vi "Ergetization.vi"(8 "error in (no error)":errorcluster, 11 "Maze in":refnum<class "Maze.lvclass">) -> (0 "error out":errorcluster, 2 "size":i32, 3 "Maze out":refnum<class "Maze.lvclass">)   [LabVIEW 2021, in "Maze.lvclass"]
uses:
  Maze.lvclass
  Maze.lvclass/Maze.ctl
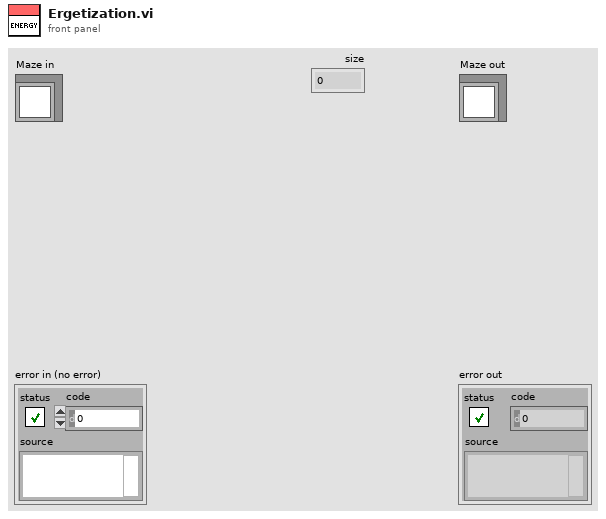
[diagram p1: front panel]
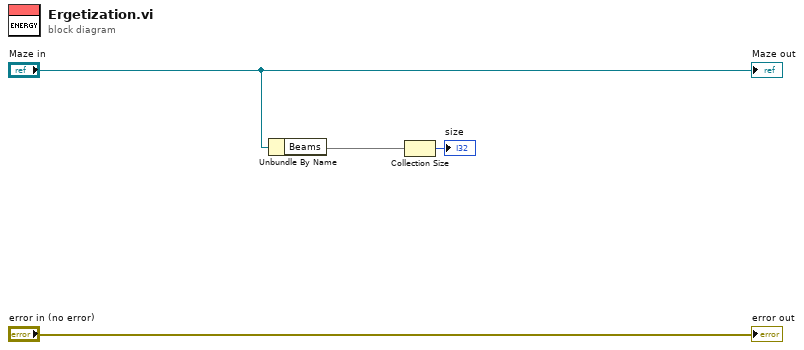
[diagram p0: block diagram]
diagram:
  n1 = Unbundle By Name("Maze in") -> ("Beams"=w2:set{refnum<class "Beam.lvclass">})
  n2 = Collection Size(1:w2) -> (0:→"size":i32)
  "error out" <- "error in (no error)"
  "Maze out" <- "Maze in"
